vi "Main.vi"(10 "Monedas subpanel":refnum<vi>, 11 "Module Admin":refnum<class "Delacor_lib_QMH_Module Admin.lvclass">) -> ()   [LabVIEW 2020, in "Monedas.lvlib"]
doc: "This template is based off of the Queued Message Handler design pattern and the Queued Message Handler project template that ships with LabVIEW.\n\nThe main difference is that the queue is private to this module and communication between modules is performed via Broadcast and Request events.\n\nRequest events are wrapped in public API methods and are handled in the Event Handling Loop (EHL) of this VI. Any module can register for Broadcast events sent by this module. The EHL generates messages based on user interface actions.\n\nThe Message Handling Loop (MHL) processes messages generated by the EHL, or by other messages. The messages are string values, so new messages can be added easily to the Message Cases case structure in the MHL. Each message cluster can also provide an optional value for Message Data, which is a variant that can be converted to whatever message-specific data is required.\n_____\nBased on Delacor QMH Project Template 5.0.0.82."
uses:
  Monedas.lvlib
  <vilib>/Delacor/Delacor QMH/Libraries/Module Admin_class/Delacor_lib_QMH_Module Admin.lvclass
  Module Data--cluster.ctl
  Stop Argument--cluster.ctl
  <vilib>/Delacor/Delacor QMH/Libraries/Message Queue_class/Delacor_lib_QMH_Message Queue.lvclass/Delacor_lib_QMH_Message Queue.ctl
  <vilib>/Delacor/Delacor QMH/Libraries/Module Admin_class/Delacor_lib_QMH_Module Admin.lvclass/Delacor_lib_QMH_Module Admin.ctl
  Obtain config Argument--cluster.ctl
  compras Argument--cluster.ctl
  <vilib>/Utility/miscctls.llb/LVPointTypeDef.ctl
  <vilib>/Delacor/Delacor QMH/Libraries/Message Queue_class/Delacor_lib_QMH_Enqueue Message (Single).vi
  <vilib>/Delacor/Delacor QMH/Libraries/Module Admin_class/Delacor_lib_QMH_Get External Launch.vi
  <vilib>/Utility/error.llb/Error Cluster From Error Code.vi
  <vilib>/ErrorRing/Error Ring.xnode
  <vilib>/Delacor/Delacor QMH/Libraries/Message Queue_class/Delacor_lib_QMH_Message Queue.lvclass
  Mensajes/Mensajes.lvlib
  Productos/Productos.lvlib
panel:
  in  "?":T1
  out "error out":errorcluster
  out "Status":string
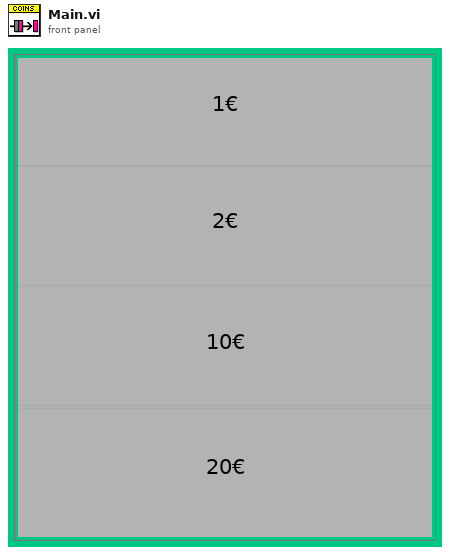
[diagram p1: front panel]
types:
  T1 = cluster{"B1":bool, "B2":bool, "B3":bool, "B4":bool}
  T2 = typedef "Monedas.lvlib/Request Events--cluster.ctl" = cluster{"Stop Module":refnum<user-event>, "Show Panel":refnum<user-event>, "Hide Panel":refnum<user-event>, "Get Module Execution Status":refnum<user-event>, "Show Diagram":refnum<user-event>, "Read Config":refnum<user-event>, "Obtain config":refnum<user-event>, "write config":refnum<user-event>, "compras":refnum<user-event>}
  T3 = typedef "Monedas.lvlib/Module Data--cluster.ctl" = cluster{"Monedas":cluster{"Denominacion1":string, "Valor":dbl, "Denominacion2":string, "Valor 2":dbl, "Denominacion3":string, "Valor 3":dbl, "Denominacion4":string, "Valor 4":dbl}}
  T4 = enum32{"invalid lock state", "Not Locked", "Locked (No Password)", "Password-protected"}
  T5 = typedef "Monedas.lvlib/Stop Argument--cluster.ctl" = cluster{"Origin":string, "Exit via Stop Module Req?":bool, "Wait for Module to stop?":bool}
  T6 = typedef "Monedas.lvlib/compras Argument--cluster.ctl" = cluster{"Numeric":dbl, "Boolean":bool}
  T7 = typedef "LVPointTypeDef.ctl" = cluster{"Horizontal":i16, "Vertical":i16}
  T8 = enum32{"Invalid", "Standard", "Closed", "Hidden", "Minimized", "Maximized"}
  T9 = typedef "Monedas.lvlib/Obtain config Argument--cluster.ctl" = cluster{"Monedas 3":cluster{"Denominacion1":string, "Valor":dbl, "Denominacion2":string, "Valor 2":dbl, "Denominacion3":string, "Valor 3":dbl, "Denominacion4":string, "Valor 4":dbl}}
  T10 = cluster{"Denominacion1":string, "Valor":dbl, "Denominacion2":string, "Valor 2":dbl, "Denominacion3":string, "Valor 3":dbl, "Denominacion4":string, "Valor 4":dbl}[]
  T11 = cluster{"Monedas 2[0]":cluster{"Denominacion1":string, "Valor":dbl, "Denominacion2":string, "Valor 2":dbl, "Denominacion3":string, "Valor 3":dbl, "Denominacion4":string, "Valor 4":dbl}, "Monedas 2[1]":cluster{"Denominacion1":string, "Valor":dbl, "Denominacion2":string, "Valor 2":dbl, "Denominacion3":string, "Valor 3":dbl, "Denominacion4":string, "Valor 4":dbl}, "Monedas 2[2]":cluster{"Denominacion1":string, "Valor":dbl, "Denominacion2":string, "Valor 2":dbl, "Denominacion3":string, "Valor 3":dbl, "Denominacion4":string, "Valor 4":dbl}, "Monedas 2[3]":cluster{"Denominacion1":string, "Valor":dbl, "Denominacion2":string, "Valor 2":dbl, "Denominacion3":string, "Valor 3":dbl, "Denominacion4":string, "Valor 4":dbl}, "Monedas 2[4]":cluster{"Denominacion1":string, "Valor":dbl, "Denominacion2":string, "Valor 2":dbl, "Denominacion3":string, "Valor 3":dbl, "Denominacion4":string, "Valor 4":dbl}, "Monedas 2[5]":cluster{"Denominacion1":string, "Valor":dbl, "Denominacion2":string, "Valor 2":dbl, "Denominacion3":string, "Valor 3":dbl, "Denominacion4":string, "Valor 4":dbl}, "Monedas 2[6]":cluster{"Denominacion1":string, "Valor":dbl, "Denominacion2":string, "Valor 2":dbl, "Denominacion3":string, "Valor 3":dbl, "Denominacion4":string, "Valor 4":dbl}, "Monedas 2[7]":cluster{"Denominacion1":string, "Valor":dbl, "Denominacion2":string, "Valor 2":dbl, "Denominacion3":string, "Valor 3":dbl, "Denominacion4":string, "Valor 4":dbl}, "Monedas 2[8]":cluster{"Denominacion1":string, "Valor":dbl, "Denominacion2":string, "Valor 2":dbl, "Denominacion3":string, "Valor 3":dbl, "Denominacion4":string, "Valor 4":dbl}}
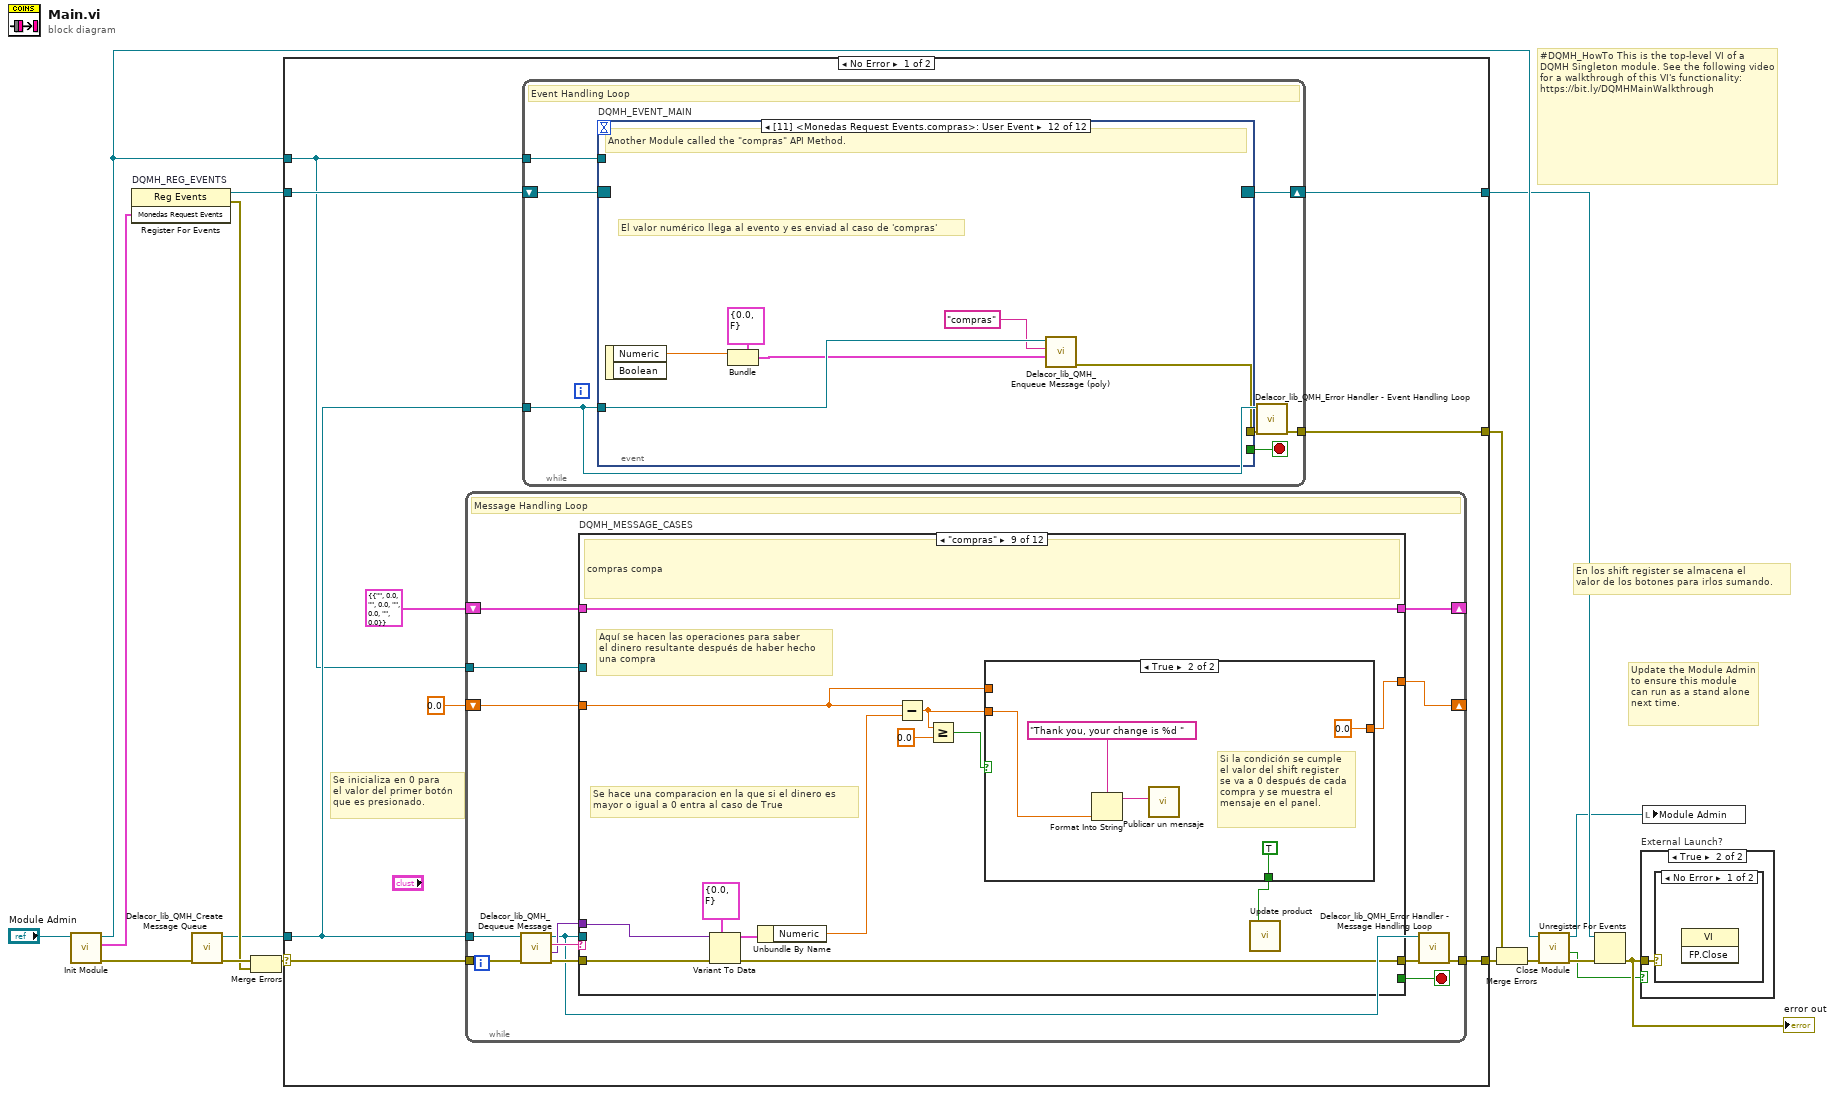
[diagram p0: block diagram]
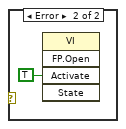
[diagram p3: hidden frame]
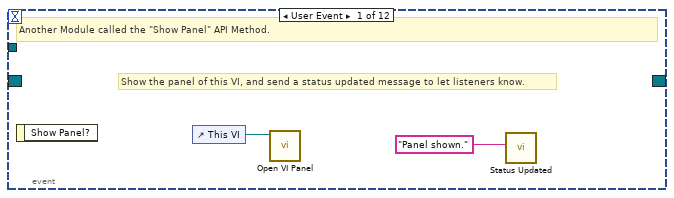
[diagram p4: hidden frame]
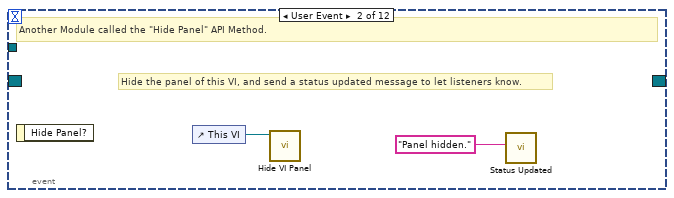
[diagram p5: hidden frame]
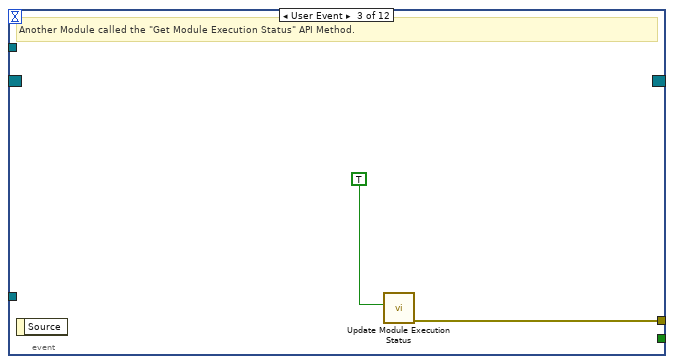
[diagram p6: hidden frame]
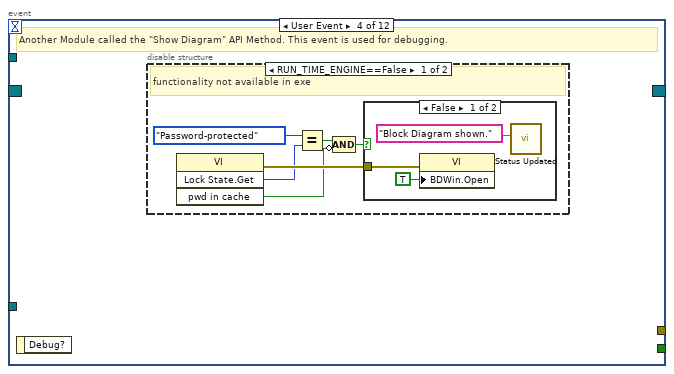
[diagram p7: hidden frame]
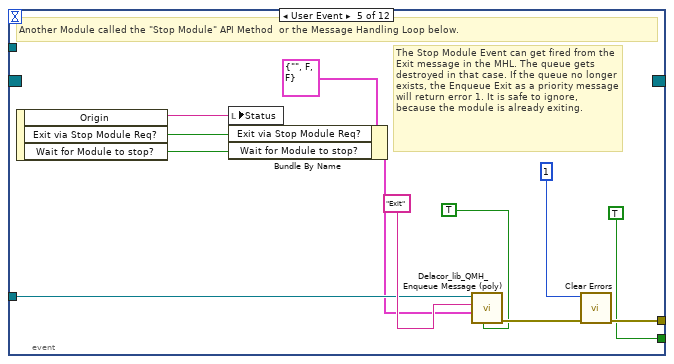
[diagram p10: hidden frame]
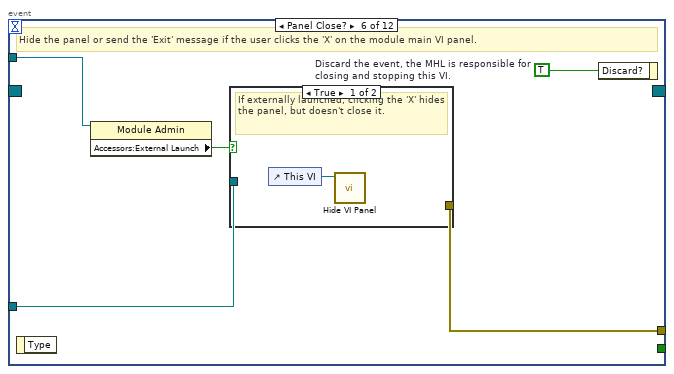
[diagram p11: hidden frame]
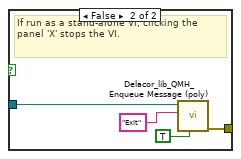
[diagram p12: hidden frame]
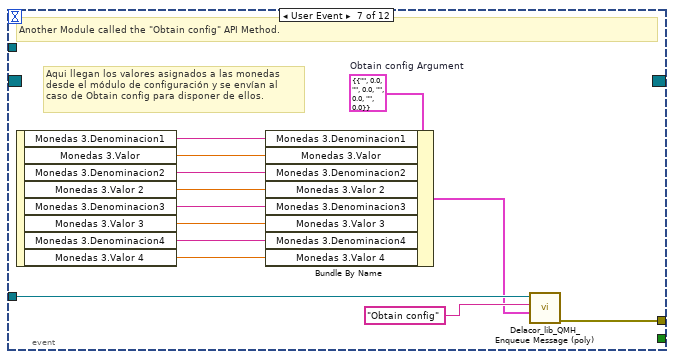
[diagram p13: hidden frame]
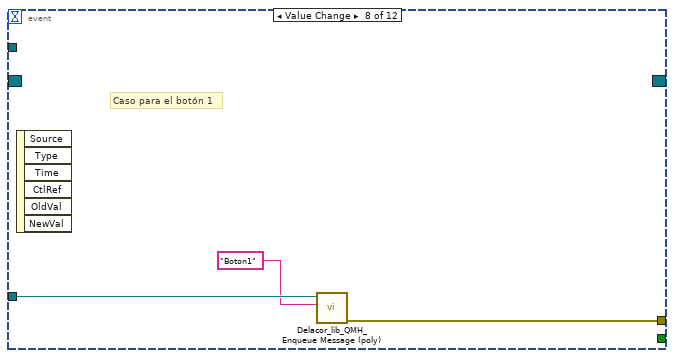
[diagram p14: hidden frame]
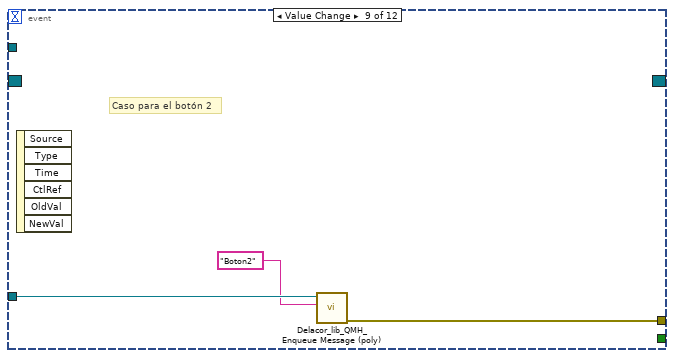
[diagram p15: hidden frame]
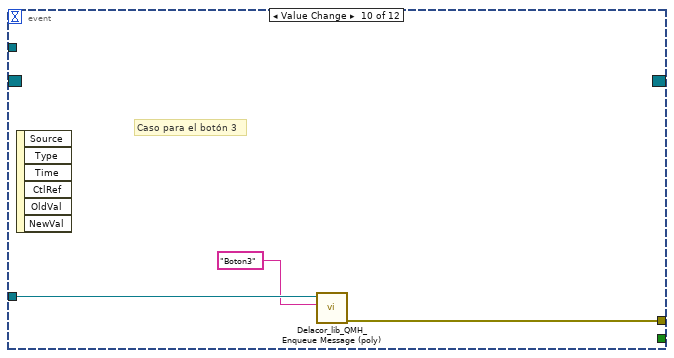
[diagram p16: hidden frame]
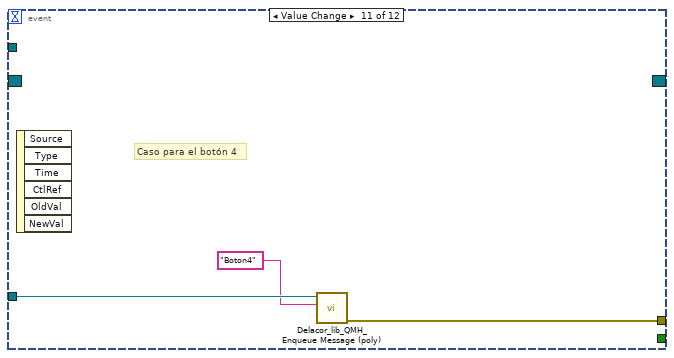
[diagram p17: hidden frame]
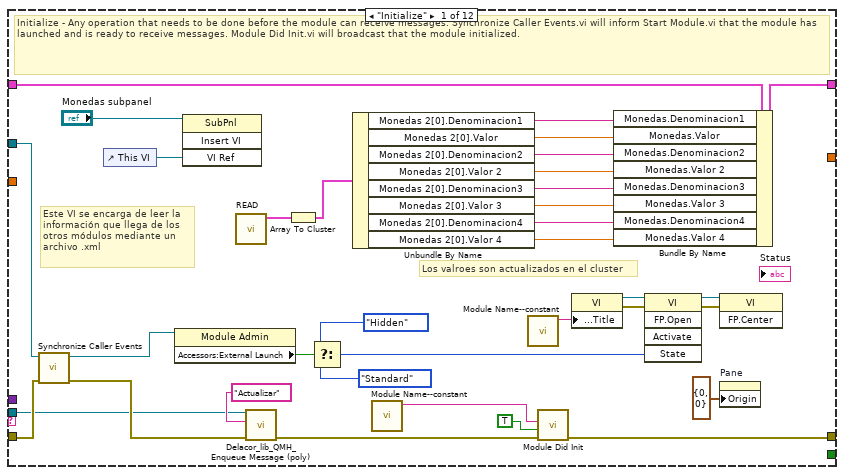
[diagram p18: hidden frame]
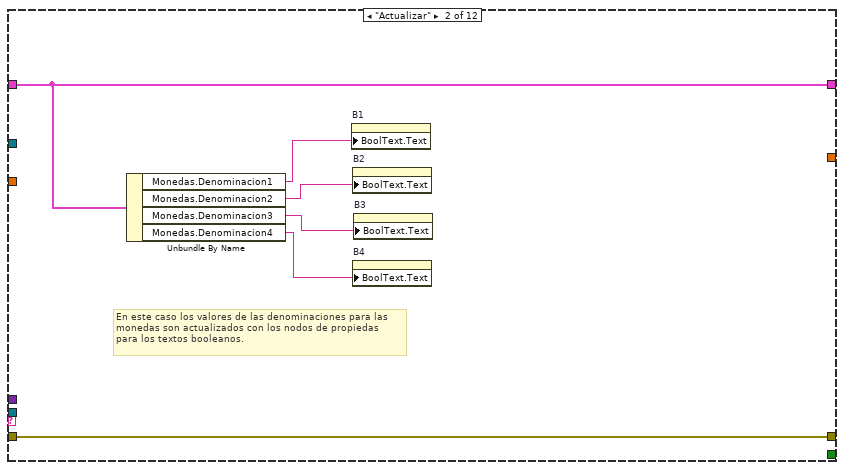
[diagram p19: hidden frame]
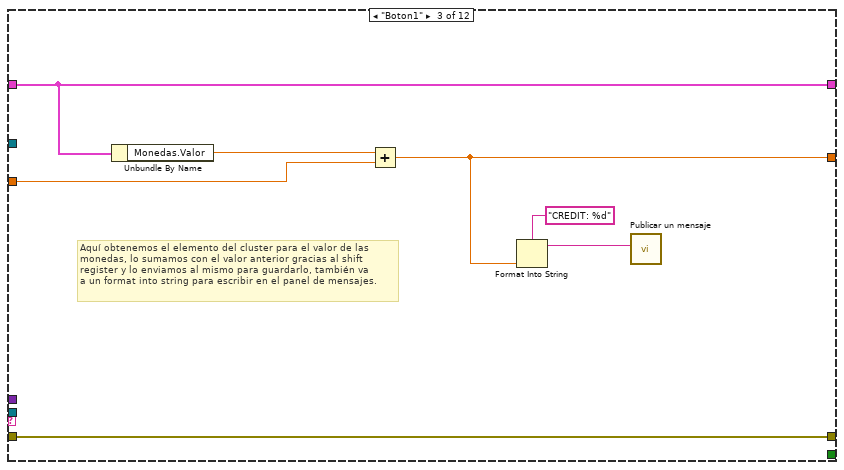
[diagram p20: hidden frame]
diagram:
  # "En los shift register se almacena el \nvalor de los botones para irlos sumando."
  # "#DQMH_HowTo This is the top-level VI of a DQMH Singleton module. See the following video for a walkthrough of this VI's functionality: https://bit.ly/DQMHMainWalkthrough"
  # "Update the Module Admin to ensure this module can run as a stand alone next time."
  n1 = call "Init Module.vi"("Singleton Module Admin in"="Module Admin") -> ("error out"=w16:errorcluster, "Monedas Request Events"=w5:T2, "Singleton Module Admin out"=w8:refnum<class "Delacor_lib_QMH_Module Admin.lvclass">)  [unwired: 8 in]
  n2 = register-events "DQMH_REG_EVENTS"(w5) -> (reference out=w6:refnum<event-registration>, error out=w9:errorcluster)  [unwired: 2 in]
  n3 = call <vilib>:"Delacor_lib_QMH_Create Message Queue.vi"("error in (no error)"=w16) -> ("error out"=w11:errorcluster, "Message Queue"=w4:refnum<class "Delacor_lib_QMH_Message Queue.lvclass">)  [unwired: 9 in]
  n4 = Merge Errors(w11, w9) -> (w10:errorcluster)
  n5 = case shown="No Error" w10 {
    selector: w10 -> [w24 w281]
    tunnel: [w26 w280] -> w17
    tunnel: [w23 w286] -> w7
    tunnel: w6 -> [w21 w286]
    tunnel: w4 -> [w20 w279]
    tunnel: [w25 _] -> w14
    tunnel: w8 -> [w19 w282]
    frame No Error {
      # "Se inicializa en 0 para\nel valor del primer botón\nque es presionado."
      n6 = while {
        tunnel: w20 -> [w106]
        shift-right: [w110] -> _
        shift-left: T3 {"Monedas"={"Denominacion1"="", "Valor"=0.0, "Denominacion2"="", "Valor 2"=0.0, "Denominacion3"="", "Valor 3"=0.0, "Denominacion4"="", "Valor 4"=0.0}} ("Data Cluster") -> [w111]
        tunnel: w24 -> [w114]
        tunnel: [w112] -> w26
        tunnel: w19 -> [w104]
        shift-right: [w103] -> _
        shift-left: 0.0 -> [w102]
        stop <- w109 stop-if-true
        # "Message Handling Loop"
        n7 = call-dynamic "Delacor_lib_QMH_Dequeue Message.vi"("error in (no error)"=w114, "Message Queue in"=w106) -> ("error out"=w113:errorcluster, "Message Data"=w107:variant, "Message"=w108:string, "Message Queue out"=w105:refnum<class "Delacor_lib_QMH_Message Queue.lvclass">)  [unwired: 6 in]
        n8 = case "DQMH_MESSAGE_CASES" shown="\"compras\"" w108 {
          selector: w108 -> [_ _ _ _ _ _ _ _ _ _ _ w266]
          tunnel: w105 -> [w126 _ _ _ _ _ w189 w207 _ w236 w258 _]
          tunnel: w113 -> [w147 w155 w156 w169 w176 w183 w191 w209 w223 w243 w264 w268]
          tunnel: [w146 w155 w156 w169 w176 w183 w187 w208 w221 w239 w261 w269] -> w115
          tunnel: w111 -> [w137 w154 w162 w168 w175 w182 w184 w206 w222 w238 w257 w267]
          tunnel: [w136 w154 w162 w168 w175 w182 w184 w205 w222 w238 w257 w267] -> w110
          tunnel: [_ _ _ _ _ _ _ _ _ _ w256 _] -> w109
          tunnel: w107 -> [_ _ _ _ _ _ w194 _ w213 w237 w255 _]
          tunnel: w104 -> [w138 _ _ _ _ _ _ _ _ w235 w250 _]
          tunnel: [_ _ w157 w163 w170 w177 _ _ w216 _ _ _] -> w103
          tunnel: w102 -> [_ _ w160 w166 w173 w180 _ _ w215 _ _ _]
          frame "Initialize" {
            # "Los valroes son actualizados en el cluster"
            # "Este VI se encarga de leer la\ninformación que llega de los\notros módulos mediante un \narchivo .xml"
            # "Initialize - Any operation that needs to be done before the module can receive messages. Synchronize Caller Events.vi will inform Start Module.vi that the module has launched and is ready to receive messages. Module Did Init.vi will broadcast that the module initialized."
            n9 = call "Synchronize Caller Events.vi"("error in (no error)"=w147, "Singleton Module Admin in"=w138) -> ("error out"=w128:errorcluster, "Singleton Module Admin out"=w133:refnum<class "Delacor_lib_QMH_Module Admin.lvclass">)  [unwired: 8 in]
            n10 = control-ref of="This VI"() -> (w130:refnum<vi>)
            n11 = property class="Module Admin"(reference=w133) -> ("Accessors:External Launch"=w142:bool)  [unwired: 1 in, 2 out]
            n12 = invoke class="SubPnl" method="Insert VI"(reference="Monedas subpanel", "VI Ref"=w130) -> ()  [unwired: 2 in, 4 out]
            n13 = call "READ.vi"() -> ("Monedas 2"=w117:T10)  [unwired: 10 in, 1 out]
            n14 = call-poly <vilib>:"Delacor_lib_QMH_Enqueue Message (poly).vi"("error in (no error)"=w128, "Message"="Actualizar", "Message Queue in"=w126) -> ("error out"=w127:errorcluster)  [unwired: 7 in, 1 out]
            n15 = Array To Cluster(array=w117) -> (cluster=w116:T11)
            n16 = Select(t=T8."Hidden" ("State"), s=w142, f=T8."Standard" ("State")) -> (s? t:f=w139:T8)
            n17 = Unbundle By Name(w116) -> ("Monedas 2[0].Denominacion1"=w125:string, "Monedas 2[0].Valor"=w124:dbl, "Monedas 2[0].Denominacion2"=w123:string, "Monedas 2[0].Valor 2"=w122:dbl, "Monedas 2[0].Denominacion3"=w121:string, "Monedas 2[0].Valor 3"=w120:dbl, "Monedas 2[0].Denominacion4"=w119:string, "Monedas 2[0].Valor 4"=w118:dbl)
            n18 = call "Module Name--constant.vi"() -> ("Module Name"=w134:string)  [unwired: 11 in]
            n19 = call "Module Name--constant.vi"() -> ("Module Name"=w145:string)  [unwired: 11 in]
            n20 = call "Module Did Init.vi"("error in (no error)"=w127, "Initialized?"=TRUE, "Origin"=w134) -> ("error out"=w146:errorcluster)  [unwired: 8 in]
            n21 = property class="VI"("Front Panel.Title"=w145) -> (reference out=w144:refnum<vi>, error out=w149:errorcluster)  [unwired: 2 in]
            n22 = Bundle By Name(cluster=w137, "Monedas.Denominacion1"=w125, "Monedas.Valor"=w124, "Monedas.Denominacion2"=w123, "Monedas.Valor 2"=w122, "Monedas.Denominacion3"=w121, "Monedas.Valor 3"=w120, "Monedas.Denominacion4"=w119, "Monedas.Valor 4"=w118) -> (w136:T3)
            n23 = invoke class="VI" method="FP.Open"(reference=w144, error in=w149, "State"=w139) -> (reference out=w143:refnum<vi>, error out=w148:errorcluster)  [unwired: 2 in, 3 out]
            n24 = invoke class="VI" method="FP.Center"(reference=w143, error in=w148) -> ()  [unwired: 1 in, 3 out]
            n25 = property on="Pane" class="Pane"("Origin"=T7 {"Horizontal"=0, "Vertical"=0}) -> ()  [unwired: 2 in, 2 out]
          }
          frame "Actualizar" {
            # "En este caso los valores de las denominaciones para las\nmonedas son actualizados con los nodos de propiedas\npara los textos booleanos."
            n26 = Unbundle By Name(w154) -> ("Monedas.Denominacion1"=w153:string, "Monedas.Denominacion2"=w152:string, "Monedas.Denominacion3"=w151:string, "Monedas.Denominacion4"=w150:string)
            n27 = property on="B1" class="Bool"("BoolText.Text"=w153) -> ()  [unwired: 2 in, 2 out]
            n28 = property on="B2" class="Bool"("BoolText.Text"=w152) -> ()  [unwired: 2 in, 2 out]
            n29 = property on="B4" class="Bool"("BoolText.Text"=w150) -> ()  [unwired: 2 in, 2 out]
            n30 = property on="B3" class="Bool"("BoolText.Text"=w151) -> ()  [unwired: 2 in, 2 out]
          }
          frame "Boton1" {
            # "Aquí obtenemos el elemento del cluster para el valor de las \nmonedas, lo sumamos con el valor anterior gracias al shift\nregister y lo enviamos al mismo para guardarlo, también va \na un format into string para escribir en el panel de mensajes."
            n31 = Unbundle By Name(w162) -> ("Monedas.Valor"=w161:dbl)
            n32 = Add(x=w161, y=w160) -> (x+y=w157:dbl)
            n33 = Format Into String(format string="CREDIT: %d", w157) -> (resulting string=w158:string)  [unwired: 2 in, 1 out]
            n34 = call "Publicar un mensaje.vi"("Mensaje"=w158) -> ()  [unwired: 10 in, 1 out]
          }
          frame "Boton2" {
            # "Lo mismo para los cuatro botones"
            n35 = Unbundle By Name(w168) -> ("Monedas.Valor 2"=w167:dbl)
            n36 = Add(x=w167, y=w166) -> (x+y=w163:dbl)
            n37 = Format Into String(format string="CREDIT: %d", w163) -> (resulting string=w165:string)  [unwired: 2 in, 1 out]
            n38 = call "Publicar un mensaje.vi"("Mensaje"=w165) -> ()  [unwired: 10 in, 1 out]
          }
          frame "Boton3" {
            n39 = Unbundle By Name(w175) -> ("Monedas.Valor 3"=w174:dbl)
            n40 = Add(x=w174, y=w173) -> (x+y=w170:dbl)
            n41 = Format Into String(format string="CREDIT: %d", w170) -> (resulting string=w172:string)  [unwired: 2 in, 1 out]
            n42 = call "Publicar un mensaje.vi"("Mensaje"=w172) -> ()  [unwired: 10 in, 1 out]
          }
          frame "Boton4" {
            n43 = Unbundle By Name(w182) -> ("Monedas.Valor 4"=w181:dbl)
            n44 = Add(x=w181, y=w180) -> (x+y=w177:dbl)
            n45 = Format Into String(format string="CREDIT: %d", w177) -> (resulting string=w179:string)  [unwired: 2 in, 1 out]
            n46 = call "Publicar un mensaje.vi"("Mensaje"=w179) -> ()  [unwired: 10 in, 1 out]
          }
          frame "Obtain config" {
            # "Aqui los valores se van al VI de write y posteriormente a Leer\npara ser actualizados en el cluster con el VI de leer de nuevo"
            # "This event obtain the info from the config. module"
            n47 = call-poly <vilib>:"Delacor_lib_QMH_Enqueue Message (poly).vi"("error in (no error)"=w191, "Message"="Leer", "Message Queue in"=w189) -> ("error out"=w190:errorcluster)  [unwired: 7 in, 1 out]
            n48 = Variant To Data(error in=w190, type=T9 {"Monedas 3"={"Denominacion1"="", "Valor"=0.0, "Denominacion2"="", "Valor 2"=0.0, "Denominacion3"="", "Valor 3"=0.0, "Denominacion4"="", "Valor 4"=0.0}} ("Obtain config Argument"), Variant=w194) -> (data=w186:T9, error out=w188:errorcluster)
            n49 = Cluster To Array(cluster=w186) -> (array=w185:T10)
            n50 = call "WRITE.vi"("error in (no error)"=w188, "Monedas 3"=w185) -> ("error out"=w187:errorcluster)  [unwired: 9 in]
          }
          frame "Leer" {
            # "Aqui los valores se llen desde el archiv .xml y se suben al cluster"
            # "This event obtain the info from the config. module"
            n51 = call "READ.vi"() -> ("Monedas 2"=w204:T10)  [unwired: 10 in, 1 out]
            n52 = Array To Cluster(array=w204) -> (cluster=w203:T11)
            n53 = call-poly <vilib>:"Delacor_lib_QMH_Enqueue Message (poly).vi"("error in (no error)"=w209, "Message"="Actualizar", "Message Queue in"=w207) -> ("error out"=w208:errorcluster)  [unwired: 7 in, 1 out]
            n54 = Unbundle By Name(w203) -> ("Monedas 2[0].Denominacion1"=w202:string, "Monedas 2[0].Valor"=w201:dbl, "Monedas 2[0].Denominacion2"=w200:string, "Monedas 2[0].Valor 2"=w199:dbl, "Monedas 2[0].Denominacion3"=w198:string, "Monedas 2[0].Valor 3"=w197:dbl, "Monedas 2[0].Denominacion4"=w196:string, "Monedas 2[0].Valor 4"=w195:dbl)
            n55 = Bundle By Name(cluster=w206, "Monedas.Denominacion1"=w202, "Monedas.Valor"=w201, "Monedas.Denominacion2"=w200, "Monedas.Valor 2"=w199, "Monedas.Denominacion3"=w198, "Monedas.Valor 3"=w197, "Monedas.Denominacion4"=w196, "Monedas.Valor 4"=w195) -> (w205:T3)
          }
          frame "compras" {
            # "Se hace una comparacion en la que si el dinero es \nmayor o igual a 0 entra al caso de True"
            # "Aquí se hacen las operaciones para saber\nel dinero resultante después de haber hecho\nuna compra"
            # "compras compa"
            n56 = Variant To Data(error in=w223, type=T6 {"Numeric"=0.0, "Boolean"=FALSE} ("compras Argument"), Variant=w213) -> (data=w219:T6, error out=w221:errorcluster)
            n57 = Unbundle By Name(w219) -> ("Numeric"=w218:dbl)
            n58 = Subtract(x=w215, y=w218) -> (x-y=w214:dbl)
            n59 = Greater Or Equal?(x=w214, y=0.0) -> (x >= y?=w212:bool)
            n60 = case shown="True" w212 {
              tunnel: [w227 0.0] -> w216
              tunnel: w215 -> [w227 _]
              tunnel: w214 -> [_ w231]
              tunnel: [FALSE ("enable") TRUE ("enable")] -> w211
              frame False {
                # "Si la condicion no va, se escribe el mensaje y el \nUpdate product se pone en falso. este evento contiene un booleando que se activa o no."
                n61 = Format Into String(format string="Need more credit, you have   %d" ("Mensaje"), w227) -> (resulting string=w225:string)  [unwired: 2 in, 1 out]
                n62 = call "Publicar un mensaje.vi"("Mensaje"=w225) -> ()  [unwired: 10 in, 1 out]
              }
              frame True {
                # "Si la condición se cumple\nel valor del shift register \nse va a 0 después de cada\ncompra y se muestra el\nmensaje en el panel."
                n63 = Format Into String(format string="Thank you, your change is %d " ("Mensaje"), w231) -> (resulting string=w229:string)  [unwired: 2 in, 1 out]
                n64 = call "Publicar un mensaje.vi"("Mensaje"=w229) -> ()  [unwired: 10 in, 1 out]
              }
            }
            n65 = call "Update product.vi"("enable"=w211) -> ()  [unwired: 10 in, 1 out]
          }
          frame "Error" {
            # "Error - Check the error message data and respond accordingly. This message is sent by the \"Error Handler\" VIs at the end of each loop in this application."
            n66 = Variant To Data(error in=w243, type=errorcluster {"status"=FALSE, "code"=0, "source"=""} ("error constant"), Variant=w237) -> (data=w244:errorcluster, error out=w241:errorcluster)
            n67 = property class="Module Admin"(reference=w235) -> ("Accessors:External Launch"=w234:bool)  [unwired: 1 in, 2 out]
            n68 = call "Module Name--constant.vi"() -> ("Module Name"=w233:string)  [unwired: 11 in]
            n69 = call "Error Reported.vi"("Additional Information"=w233, "Error"=w244) -> ()  [unwired: 9 in, 1 out]
            n70 = case shown="False" w234 {
              tunnel: [w249 _] -> w240
              tunnel: w236 -> [w247 _]
              tunnel: w244 -> [w248 _]
              frame False {
                n71 = call <vilib>:"Simple Error Handler.vi"("error in (no error)"=w248) -> ()  [unwired: 4 in, 5 out]
                n72 = call-poly <vilib>:"Delacor_lib_QMH_Enqueue Message (poly).vi"("Priority Message? (F)"=TRUE, "Message"="Exit", "Message Queue in"=w247) -> ("error out"=w249:errorcluster)  [unwired: 7 in, 1 out]
              }
              frame True {
                # "If the module was launched externally, calling the Error Reported broadcast VI is the only action performed by the \"Error\" message. The module's caller can then process the error appropriately."
              }
            }
            n73 = Merge Errors(w241, w240) -> (w239:errorcluster)
            n74 = local write "error out"(w239) -> ()
          }
          frame "Exit" {
            w254 = 91  # 91: not all Exit messages will have an argument
            w256 = TRUE  # Stop the VI
            # "Exit - Exit the application."
            n75 = Variant To Data(error in=w264, type=T5 {"Origin"="", "Exit via Stop Module Req?"=FALSE, "Wait for Module to stop?"=FALSE} ("Stop Argument"), Variant=w255) -> (data=w252:T5, error out=w260:errorcluster)
            n76 = call <vilib>:"Clear Errors.vi"("error in (no error)"=w260, "specific error code to clear (0: all)"=w254) -> ("error out"=w263:errorcluster)  [unwired: 4 in, 1 out]
            n77 = control-ref of="This VI"() -> (w251:refnum<vi>)
            n78 = call-dynamic "Delacor_lib_QMH_Release Message Queue.vi"("error in (no error)"=w263, "Message Queue"=w258) -> ("error out"=w262:errorcluster)  [unwired: 9 in]
            n79 = call "Handle Exit.vi"("Stop Argument"=w252, "Admin in"=w250, "VI reference"=w251) -> ("error out"=w259:errorcluster)  [unwired: 7 in, 1 out]
            n80 = Merge Errors(w262, w259) -> (w261:errorcluster)
          }
          frame Default {
            # "'Default' case only runs if there is a message that isn't defined in any of the other cases.  Output a programming error."
            n81 = call "Module Name--constant.vi"() -> ("Module Name"=w265:string)  [unwired: 11 in]
            n82 = xnode "Error Ring"("parameter 0"=w266, "parameter 1"=w265) -> ("error out"=w270:errorcluster)
            n83 = Merge Errors(w268, w270) -> (w269:errorcluster)
          }
        }
        n84 = call-dynamic "Delacor_lib_QMH_Error Handler - Message Handling Loop.vi"("error in (no error)"=w115, "Message Queue in"=w105) -> ("dup error in"=w112:errorcluster)  [unwired: 8 in, 1 out]
      }
      n85 = while {
        tunnel: w20 -> [w27]
        shift-right: [w30] -> w23
        shift-left: w21 -> [w31]
        tunnel: [w32] -> w25
        tunnel: w19 -> [w28]
        stop <- w29 stop-if-true
        # "Event Handling Loop"
        n86 = event "DQMH_EVENT_MAIN" shown="[11] <Monedas Request Events.compras>: User Event" {
          selector: w31 -> [_ _ _ _ _ _ _ _ _ _ _ _]
          dyn-events: [_ _ _ _ _ _ _ _ _ _ _ _] -> w30
          timeout: _ -> [_ _ _ _ _ _ _ _ _ _ _ _]
          tunnel: [_ _ _ _ TRUE ("Discard?") _ _ _ _ _ _ _] -> w29
          tunnel: w27 -> [_ _ _ _ w56 w63 w83 w85 w88 w91 w94 w101]
          tunnel: [_ _ w39 _ w59 w65 w79 w86 w89 w92 w95 w96] -> w33
          tunnel: w28 -> [_ _ _ _ _ w62 _ _ _ _ _ _]
          event User Event {
            # "Show the panel of this VI, and send a status updated message to let listeners know."
            # "Another Module called the \"Show Panel\" API Method."
            n87 = event-data() -> ()  [unwired: 1 in, 1 out]
            n88 = control-ref of="This VI"() -> (w35:refnum<vi>)
            n89 = call "Open VI Panel.vi"("VI"=w35) -> ()  [unwired: 10 in, 1 out]
            n90 = call "Status Updated.vi"("Status"="Panel shown." ("format string")) -> ()  [unwired: 10 in, 1 out]
          }
          event User Event {
            # "Hide the panel of this VI, and send a status updated message to let listeners know."
            # "Another Module called the \"Hide Panel\" API Method."
            n91 = event-data() -> ()  [unwired: 1 in, 1 out]
            n92 = control-ref of="This VI"() -> (w37:refnum<vi>)
            n93 = call "Hide VI Panel.vi"("VI"=w37) -> ()  [unwired: 10 in, 1 out]
            n94 = call "Status Updated.vi"("Status"="Panel hidden." ("format string")) -> ()  [unwired: 10 in, 1 out]
          }
          event User Event {
            # "Another Module called the \"Get Module Execution Status\" API Method."
            n95 = event-data() -> ()  [unwired: 1 in, 1 out]
            n96 = call "Update Module Execution Status.vi"("Running?"=TRUE) -> ("error out"=w39:errorcluster)  [unwired: 10 in]
          }
          event User Event {
            # "Another Module called the \"Show Diagram\" API Method. This event is used for debugging."
            n97 = event-data() -> ()  [unwired: 1 in, 1 out]
            n98 = disable-structure shown="RUN_TIME_ENGINE==False" {
              frame condition #0 (active) {
                # "functionality not available in exe"
                n99 = invoke class="VI" method="Lock State.Get"() -> (error out=w45:errorcluster, "Get Lock State"=w44:T4, "pwd in cache"=w41:bool)  [unwired: 4 in, 1 out]
                n100 = Equal?(x=T4."Password-protected", y=w44) -> (x = y?=w42:bool)
                n101 = Compound Arithmetic op=AND(w42, invert w41) -> (w40:bool)
                n102 = case shown="False" w40 {
                  tunnel: w45 -> [w48 _]
                  frame False {
                    n103 = property class="VI"(error in=w48, "BDWin.Open"=TRUE ("Block Diagram Window:Open")) -> ()  [unwired: 1 in, 2 out]
                    n104 = call "Status Updated.vi"("Status"="Block Diagram shown." ("format string")) -> ()  [unwired: 10 in, 1 out]
                  }
                  frame True {
                    # "Password-protected VI, and the password is not in the cache. Do not show the diagram."
                  }
                }
              }
              frame condition #1 {
              }
            }
          }
          event User Event {
            # "The Stop Module Event can get fired from the Exit message in the MHL. The queue gets destroyed in that case. If the queue no longer exists, the Enqueue Exit as a priority message will return error 1. It is safe to ignore, because the module is already exiting."
            # "Another Module called the \"Stop Module\" API Method  or the Message Handling Loop below."
            n105 = event-data() -> ("Origin"=w55:string, "Exit via Stop Module Req?"=w51:bool, "Wait for Module to stop?"=w50:bool)  [unwired: 1 in]
            n106 = local write "Status"(w55) -> ()
            n107 = Bundle By Name(cluster=T5 {"Origin"="", "Exit via Stop Module Req?"=FALSE, "Wait for Module to stop?"=FALSE} ("Stop Argument"), "Exit via Stop Module Req?"=w51, "Wait for Module to stop?"=w50) -> (w49:T5)
            n108 = call-poly <vilib>:"Delacor_lib_QMH_Enqueue Message (poly).vi"("Priority Message? (F)"=TRUE, "Message Data"=w49, "Message"="Exit", "Message Queue in"=w56) -> ("error out"=w60:errorcluster)  [unwired: 6 in, 1 out]
            n109 = call <vilib>:"Clear Errors.vi"("error in (no error)"=w60, "specific error code to clear (0: all)"=1) -> ("error out"=w59:errorcluster)  [unwired: 4 in, 1 out]
          }
          event Panel Close? {
            w64 = TRUE  # Discard the event, the MHL is responsible for closing and stopping this VI.
            # "Hide the panel or send the 'Exit' message if the user clicks the 'X' on the module main VI panel."
            n110 = event-data() -> ()  [unwired: 1 in, 1 out]
            n111 = property class="Module Admin"(reference=w62) -> ("Accessors:External Launch"=w61:bool)  [unwired: 1 in, 2 out]
            n112 = case shown="True" w61 {
              tunnel: w63 -> [_ w69]
              tunnel: [_ w70] -> w65
              frame True {
                # "If externally launched, clicking the 'X' hides the panel, but doesn't close it."
                n113 = control-ref of="This VI"() -> (w66:refnum<vi>)
                n114 = call "Hide VI Panel.vi"("VI"=w66) -> ()  [unwired: 10 in, 1 out]
              }
              frame False {
                # "If run as a stand-alone VI, clicking the panel 'X' stops the VI."
                n115 = call-poly <vilib>:"Delacor_lib_QMH_Enqueue Message (poly).vi"("Priority Message? (F)"=TRUE, "Message"="Exit", "Message Queue in"=w69) -> ("error out"=w70:errorcluster)  [unwired: 7 in, 1 out]
              }
            }
            n116 = event-data("Discard?"=w64) -> ()  [unwired: 1 in, 1 out]
          }
          event User Event {
            w81 = T9 {"Monedas 3"={"Denominacion1"="", "Valor"=0.0, "Denominacion2"="", "Valor 2"=0.0, "Denominacion3"="", "Valor 3"=0.0, "Denominacion4"="", "Valor 4"=0.0}}  # Obtain config Argument
            # "Aqui llegan los valores asignados a las monedas\ndesde el módulo de configuración y se envían al \ncaso de Obtain config para disponer de ellos."
            # "Another Module called the \"Obtain config\" API Method."
            n117 = event-data() -> ("Monedas 3.Denominacion1"=w80:string, "Monedas 3.Valor"=w78:dbl, "Monedas 3.Denominacion2"=w77:string, "Monedas 3.Valor 2"=w76:dbl, "Monedas 3.Denominacion3"=w75:string, "Monedas 3.Valor 3"=w74:dbl, "Monedas 3.Denominacion4"=w73:string, "Monedas 3.Valor 4"=w72:dbl)  [unwired: 1 in]
            n118 = Bundle By Name(cluster=w81, "Monedas 3.Denominacion1"=w80, "Monedas 3.Valor"=w78, "Monedas 3.Denominacion2"=w77, "Monedas 3.Valor 2"=w76, "Monedas 3.Denominacion3"=w75, "Monedas 3.Valor 3"=w74, "Monedas 3.Denominacion4"=w73, "Monedas 3.Valor 4"=w72) -> (w71:T9)
            n119 = call-poly <vilib>:"Delacor_lib_QMH_Enqueue Message (poly).vi"("Message Data"=w71, "Message"="Obtain config", "Message Queue in"=w83) -> ("error out"=w79:errorcluster)  [unwired: 7 in, 1 out]
          }
          event Value Change {
            # "Caso para el botón 1"
            n120 = event-data() -> ()  [unwired: 1 in, 6 out]
            n121 = call-poly <vilib>:"Delacor_lib_QMH_Enqueue Message (poly).vi"("Message"="Boton1", "Message Queue in"=w85) -> ("error out"=w86:errorcluster)  [unwired: 8 in, 1 out]
          }
          event Value Change {
            # "Caso para el botón 2"
            n122 = event-data() -> ()  [unwired: 1 in, 6 out]
            n123 = call-poly <vilib>:"Delacor_lib_QMH_Enqueue Message (poly).vi"("Message"="Boton2", "Message Queue in"=w88) -> ("error out"=w89:errorcluster)  [unwired: 8 in, 1 out]
          }
          event Value Change {
            # "Caso para el botón 3"
            n124 = event-data() -> ()  [unwired: 1 in, 6 out]
            n125 = call-poly <vilib>:"Delacor_lib_QMH_Enqueue Message (poly).vi"("Message"="Boton3", "Message Queue in"=w91) -> ("error out"=w92:errorcluster)  [unwired: 8 in, 1 out]
          }
          event Value Change {
            # "Caso para el botón 4"
            n126 = event-data() -> ()  [unwired: 1 in, 6 out]
            n127 = call-poly <vilib>:"Delacor_lib_QMH_Enqueue Message (poly).vi"("Message"="Boton4", "Message Queue in"=w94) -> ("error out"=w95:errorcluster)  [unwired: 8 in, 1 out]
          }
          event User Event {
            # "El valor numérico llega al evento y es enviad al caso de 'compras'"
            # "Another Module called the \"compras\" API Method."
            n128 = event-data() -> ("Numeric"=w97:dbl)  [unwired: 1 in, 1 out]
            n129 = Bundle(cluster=T6 {"Numeric"=0.0, "Boolean"=FALSE} ("compras Argument"), "Numeric"=w97) -> (w98:T6)  [unwired: 1 in]
            n130 = call-poly <vilib>:"Delacor_lib_QMH_Enqueue Message (poly).vi"("Message Data"=w98, "Message"="compras", "Message Queue in"=w101) -> ("error out"=w96:errorcluster)  [unwired: 7 in, 1 out]
          }
        }
        n131 = call-dynamic "Delacor_lib_QMH_Error Handler - Event Handling Loop.vi"("error in (no error)"=w33, "Message Queue in"=w27) -> ("dup error in"=w32:errorcluster)  [unwired: 8 in, 1 out]
      }
    }
    frame Error {
      # "Synchronize Caller Events.vi will inform Start Module.vi that the module has launched and will let the code calling Start Module.vi register for broadcasts and would permit the caller receive the broadcast that an error occurred at launch time."
      n132 = call-dynamic "Delacor_lib_QMH_Release Message Queue.vi"("error in (no error)"=w281, "Message Queue"=w279) -> ("error out"=w280:errorcluster)  [unwired: 9 in]
      n133 = call "Synchronize Caller Events.vi"("Singleton Module Admin in"=w282) -> ("error out"=w287:errorcluster)  [unwired: 9 in, 1 out]
      n134 = call "Module Name--constant.vi"() -> ("Module Name"=w285:string)  [unwired: 11 in]
      n135 = Format Into String(format string="An error occurred during initialization. %s is no longer running.", w285) -> (resulting string=w283:string)  [unwired: 2 in, 1 out]
      n136 = Merge Errors(w280, w287) -> (w288:errorcluster)
      n137 = call "Error Reported.vi"("Additional Information"=w283, "Error"=w288) -> ()  [unwired: 9 in, 1 out]
    }
  }
  n138 = Merge Errors(w14, w17) -> (w13:errorcluster)
  n139 = call "Close Module.vi"("error in (no error)"=w13, "Module Admin in"=w8) -> ("error out"=w15:errorcluster, "External Launch"=w1:bool, "Module Admin out"=w2:refnum<class "Delacor_lib_QMH_Module Admin.lvclass">)  [unwired: 7 in]
  n140 = Unregister For Events(event registration refnum=w7, error in=w15) -> (error out=w12:errorcluster)
  "error out" <- w12
  n141 = case "External Launch?" shown="True" w1 {
    tunnel: w12 -> [_ w289]
    frame False {
    }
    frame True {
      n142 = case shown="No Error" w289 {
        frame No Error {
          n143 = invoke class="VI" method="FP.Close"() -> ()  [unwired: 3 in, 3 out]
        }
        frame Error {
          n144 = invoke class="VI" method="FP.Open"("Activate"=TRUE ("Activate?")) -> ()  [unwired: 4 in, 5 out]
        }
      }
    }
  }
  n145 = local write "Module Admin"(w2) -> ()
